vi "Post Substeps PWM Generation Task Stop.vi"(9 "PWM Output In":T1, 10 "Socket No":u16=1, 11 "Sequence Context In":refnum<k7>) -> (0 "error out":errorcluster, 3 "Report Text":string)   [LabVIEW 2023, in "LTT_TeststandSteptypes.lvlib"]
doc: "This VI Is Socket Number based AO Data Signal Write Through Q"
uses:
  LTT_TeststandSteptypes.lvlib
  HardwareAbstractionLayer_LVOOP/PWM Output/NI PWM Output_class/NI PWM DAQ/Control/PWM Output Edit.ctl
  HardwareAbstractionLayer_LVOOP/PWM Output/NI PWM Output_class/NI PWM Output.lvclass
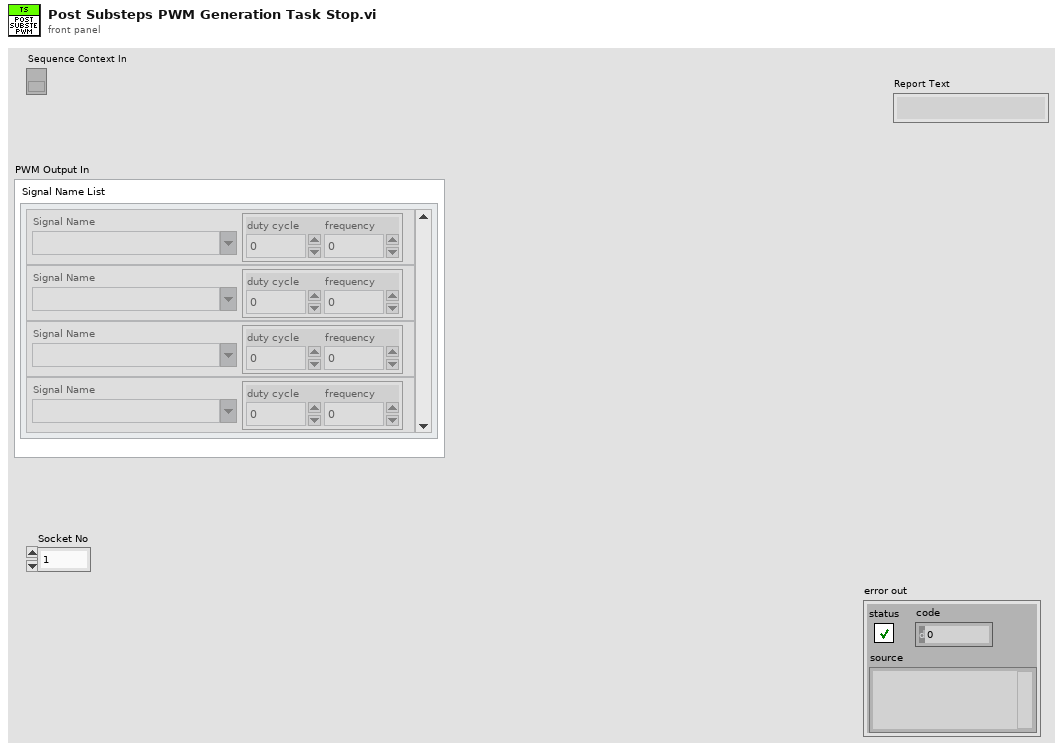
[diagram p1: front panel]
types:
  T1 = typedef "HardwareAbstractionLayer_LVOOP.lvlib/NI PWM Output.lvclass/PWM Output Edit.ctl" = cluster{"Signal Name List":cluster{"Signal Name":string, "values":cluster{"duty cycle":dbl, "frequency":dbl}}[]}
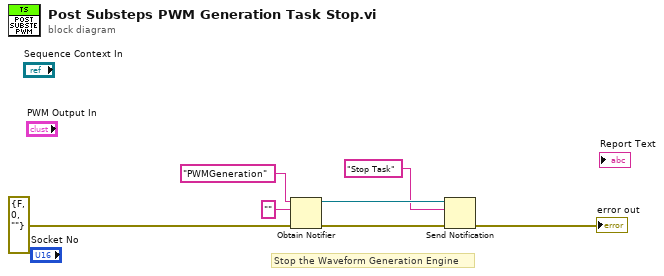
[diagram p0: block diagram]
diagram:
  # "Stop the Waveform Generation Engine"
  n1 = Obtain Notifier(name (unnamed)="PWMGeneration", notification data type="", error in (no error)=errorcluster {"status"=FALSE, "code"=0, "source"=""} ("error in")) -> (notifier out=w3:refnum<notifier>, error out=w4:errorcluster)  [unwired: 1 in, 1 out]
  n2 = Send Notification(notification="Stop Task", notifier=w3, error in (no error)=w4) -> (error out=→"error out":errorcluster)  [unwired: 1 out]
